vi "New Actor wLauncher.vi"(7 "Actor wLauncher in":refnum<class "Actor wLauncher.lvclass">, 8 "error in (no error)":errorcluster) -> (0 "error out":errorcluster, 2 "Actor's Enqueuer":refnum<class "Message Enqueuer.lvclass">, 3 "Launcher Notifier":refnum<notifier>)   [LabVIEW 2017, in "Framework.lvlib" / "Actor wLauncher.lvclass"]
uses:
  Actor wLauncher.lvclass
  C:/Program Files (x86)/National Instruments/LabVIEW 2017/vi.lib/ActorFramework/Actor/Actor.lvclass
  <vilib>/ActorFramework/Message Enqueuer/Message Enqueuer.lvclass
  Actor wLauncher.lvclass/Actor wLauncher.ctl
  <vilib>/ActorFramework/Actor/Actor.lvclass
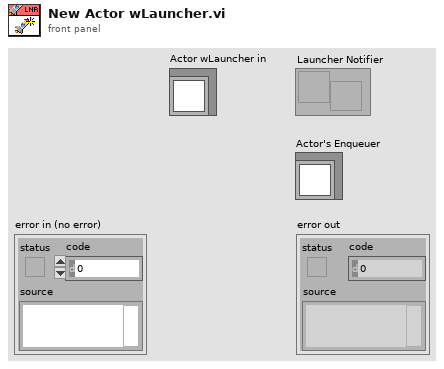
[diagram p1: front panel]
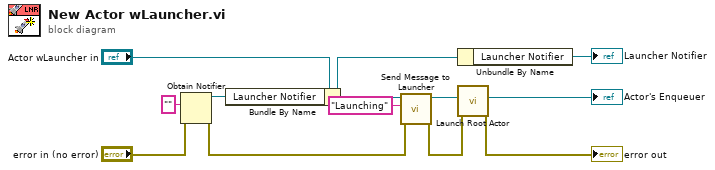
[diagram p0: block diagram]
diagram:
  n1 = Obtain Notifier(notification data type="", error in (no error)="error in (no error)") -> (notifier out=w9:refnum<notifier>, error out=w3:errorcluster)  [unwired: 2 in, 1 out]
  n2 = Bundle By Name(cluster="Actor wLauncher in", "Launcher Notifier"=w9) -> (w5:refnum<class "Actor wLauncher.lvclass">)
  n3 = call "Send Message to Launcher.vi"("error in (no error)"=w3, "Msg to Launcher"="Launching", "Actor wLauncher in"=w5) -> ("error out"=w2:errorcluster, "Actor wLauncher out"=w4:refnum<class "Actor wLauncher.lvclass">)  [unwired: 7 in]
  n4 = Unbundle By Name(w5) -> ("Launcher Notifier"=→"Launcher Notifier":refnum<notifier>)
  n5 = call <vilib>:"Launch Root Actor.vi"("error in (no error)"=w2, "Actor"=w4) -> ("error out"=→"error out":errorcluster, "Actor's Enqueuer"=→"Actor's Enqueuer":refnum<class "Message Enqueuer.lvclass">)  [unwired: 8 in]
